vi "ROSErrorCheck.vi"(2 "message":string, 3 "ROS in":T1={"topic port"=0, "Node"="", "topic"="", "type"="", "node port"=0, "error "={"status"=FALSE, "code"=0, "source"=""}, "Direction"=enum."Node", "Update (ms)"=1, "FIFO size"=1}) -> (1 "ROS out":T1={"topic port"=0, "Node"="", "topic"="", "type"="", "node port"=0, "error "={"status"=FALSE, "code"=0, "source"=""}, "Direction"=enum."Node", "Update (ms)"=1, "FIFO size"=1})   [LabVIEW 2016]
doc: "Checks for errors. Stops program if there is an error when connecting to the Master"
uses:
  SubVIs/_ROSControl.ctl
  SubVIs/_ROSDirection.ctl
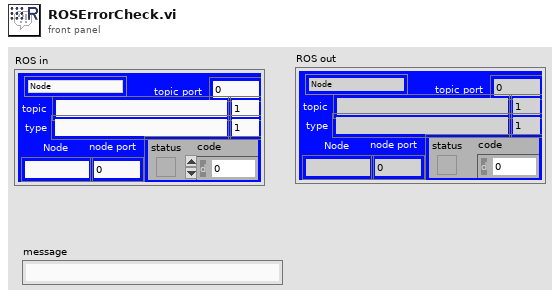
[diagram p1: front panel]
types:
  T1 = typedef "_ROSControl.ctl" = cluster{"topic port":u16, "Node":string, "topic":string, "type":string, "node port":u16, "error ":errorcluster, "Direction":T2, "Update (ms)":u16, "FIFO size":u16}
  T2 = typedef "_ROSDirection.ctl" = enum16{"Node", "Publisher", "Subscriber", "ServiceClient", "ServiceProvider"}
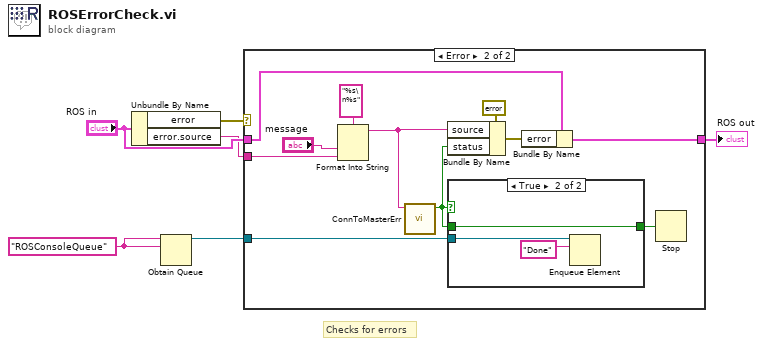
[diagram p0: block diagram]
diagram:
  w2 = "ROSConsoleQueue" ("name (unnamed)")
  # "Checks for errors"
  n1 = Unbundle By Name("ROS in") -> ("error"=w4:errorcluster, "error.source"=w3:string)
  n2 = Obtain Queue(name (unnamed)=w2, element data type=w2) -> (queue out=w1:refnum<queue>)  [unwired: 3 in, 2 out]
  n3 = case shown="Error" w4 {
    tunnel: [w7 w18] -> w6
    tunnel: "ROS in" -> [w7 w17]
    tunnel: w3 -> [_ w12]
    tunnel: w1 -> [_ w11]
    frame No Error {
    }
    frame Error {
      n4 = Format Into String(format string="%s\n%s", "message", w12) -> (resulting string=w9:string)  [unwired: 2 in, 1 out]
      n5 = call "ConnToMasterErr.vi"("String"=w9) -> ("Abort?"=w8:bool)  [unwired: 10 in]
      n6 = Bundle By Name(cluster=errorcluster {"status"=TRUE, "code"=0, "source"="Bad Topic"} ("error"), "source"=w9, "status"=w8) -> (w15:errorcluster)
      n7 = case shown="True" w8 {
        tunnel: w8 -> [_ w19]
        tunnel: w11 -> [_ w20]
        tunnel: [_ w19] -> w10
        frame False {
        }
        frame True {
          n8 = Enqueue Element(queue=w20, element="Done") -> ()  [unwired: 2 in, 3 out]
        }
      }
      n9 = Bundle By Name(cluster=w17, "error"=w15) -> (w18:T1)
      n10 = Stop(stop? (T)=w10) -> ()
    }
  }
  "ROS out" <- w6
